vi "Hatch Controller.vi"(8 "error in":errorcluster) -> ()   [LabVIEW 2018]
doc: "This VI executes continuously carrying out the current operation and responding to updates or new operations. It will often contain the timing or control code that is difficult to place directly in TeleOp. This VI generally opens all sensors and motors and isolates the rest of the robot code from knowing how the operations are carried out."
uses:
  <vilib>/Rock Robotics/WPI/Framework/Completion Status.ctl
  Hatch Setpoints.ctl
  Hatch Operations.ctl
  <vilib>/Rock Robotics/WPI/Solenoid/WPI_SolenoidChannel.ctl
  <vilib>/Rock Robotics/WPI/Solenoid/WPI_SolenoidValue.ctl
  <vilib>/Rock Robotics/WPI/Solenoid/WPI_SolenoidOpenDouble.vi
  <vilib>/Rock Robotics/WPI/Solenoid/WPI_SolenoidSetEnum.vi
  <vilib>/Rock Robotics/Network Tables/NT Write Boolean.vi
panel:
  in  "Interactive Values":T1
  out "Current\nCmd":string
  in  "Buttons":cluster{"Execute Cmd":bool, "Abort Cmd":bool}
  out "Command Timing":cluster{"Start Time (ms)":u32, "Iterations":i32}
  out "Status":T3
  # "Tip: It may be helpful to observe inputs and sensor values.\nYou may also want to display tuning or debugging controls."
  # "Interactive Command: You may fill in the settings for a command\nand schedule it with the Execute button. You can observe and abort\nany command while fine tuning the code for the controller."
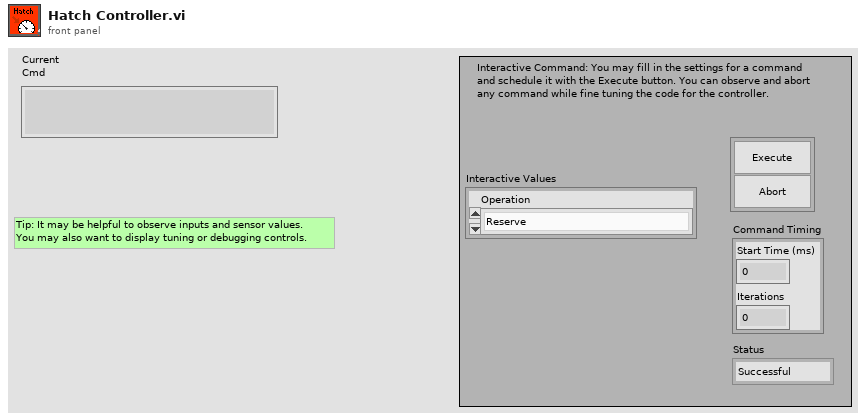
[diagram p1: front panel]
types:
  T1 = typedef "Hatch Setpoints.ctl" = cluster{"Operation":T2}
  T2 = typedef "Hatch Operations.ctl" = enum16{"Reserve", "Read Current", "Hatch Gripper In", "Hatch Gripper Out", "Extend Gripper Plate", "Retract Gripper Plate", "Retract HAB Piston", "Extend HAB Piston"}
  T3 = typedef "Completion Status.ctl" = enum16{"Successful", "Aborted", "Incomplete"}
  T4 = typedef "WPI_SolenoidChannel.ctl" = enum8{"Solenoid 0", "Solenoid 1", "Solenoid 2", "Solenoid 3", "Solenoid 4", "Solenoid 5", "Solenoid 6", "Solenoid 7", "Invalid"}
  T5 = typedef "WPI_SolenoidDevRef.ctl" = cluster{"DevStatus":errorcluster, "Pneumatics Control Module":u8, "Forward Solenoid Channel":T4, "Reverse Solenoid Channel":T4}
  T6 = typedef "Command Status Info.ctl" = cluster{"Name":string, "Status":T3, "notifier out":T7}
  T7 = typedef "Completion Notifier.ctl" = refnum<notifier>
  T8 = cluster{"Current Command":T1, "Command Timing":cluster{"Start Time (ms)":u32, "Iterations":i32}, "Command Arguments":cluster{"Command Info":T6, "Description":string, "Default Command":T1, "queue out":refnum<queue>, "Subsystem Name":string}}
  T9 = typedef "WPI_SolenoidValue.ctl" = enum16{"Off", "On", "Forward", "Reverse"}
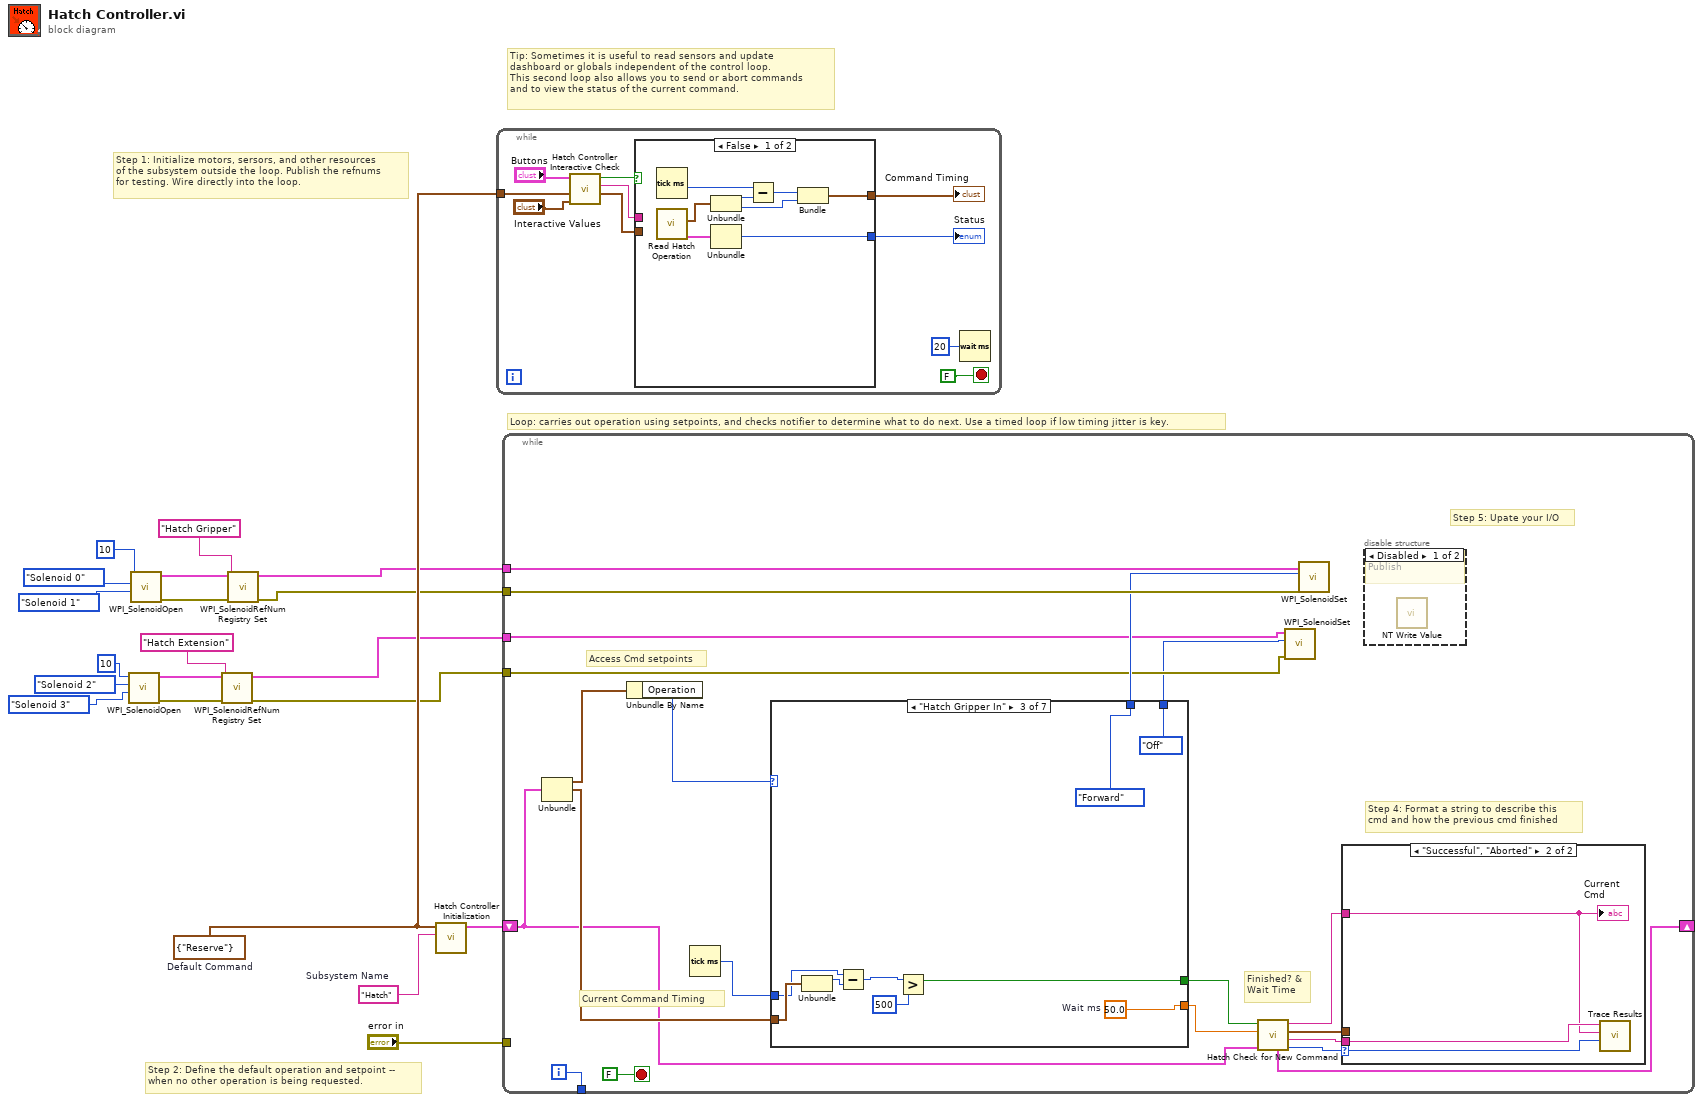
[diagram p0: block diagram]
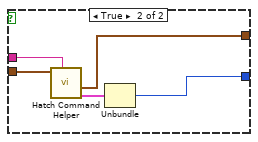
[diagram p2: hidden frame]
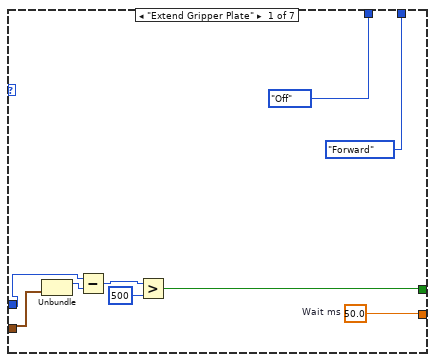
[diagram p5: hidden frame]
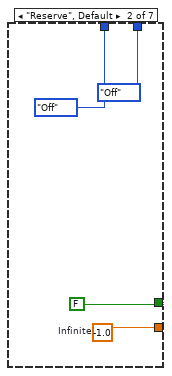
[diagram p6: hidden frame]
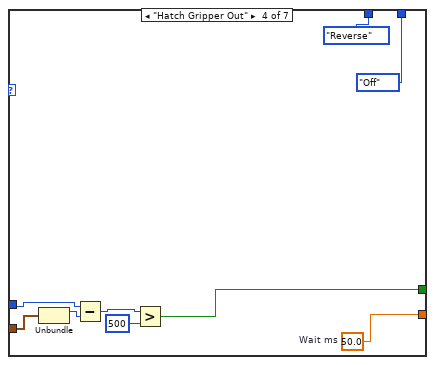
[diagram p7: hidden frame]
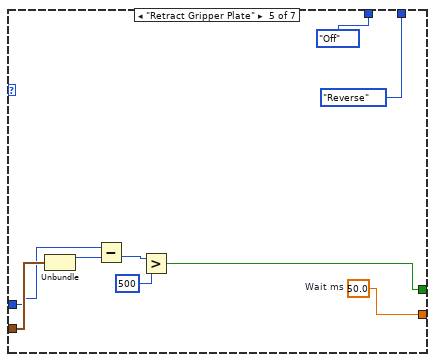
[diagram p8: hidden frame]
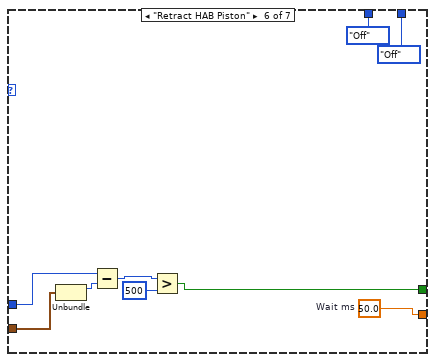
[diagram p9: hidden frame]
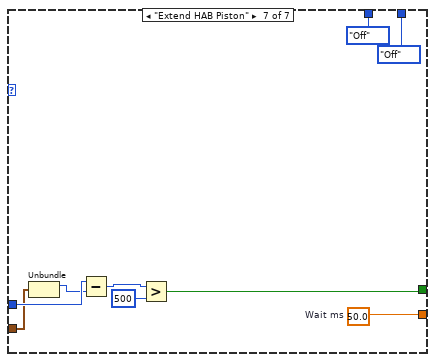
[diagram p10: hidden frame]
diagram:
  w17 = T1 {"Operation"=enum."Reserve"}  # Default Command
  w18 = "Hatch"  # Subsystem Name
  # "Tip: Sometimes it is useful to read sensors and update\ndashboard or globals independent of the control loop.\nThis second loop also allows you to send or abort commands\nand to view the status of the current command."
  # "Step 2: Define the default operation and setpoint --\nwhen no other operation is being requested."
  # "Step 1: Initialize motors, sersors, and other resources\nof the subsystem outside the loop. Publish the refnums\nfor testing. Wire directly into the loop."
  # "Loop: carries out operation using setpoints, and checks notifier to determine what to do next. Use a timed loop if low timing jitter is key."
  n1 = call-poly <vilib>:"WPI_SolenoidOpen.vi"("Reverse Solenoid Channel"=WPI_SolenoidChannel."Solenoid 3", "Forward Solenoid Channel"=WPI_SolenoidChannel."Solenoid 2", "Pneumatics Control Module (0)"=u8 10) -> ("error out"=w5:errorcluster, "SolenoidDevRef"=w4:T5)  [unwired: 7 in]
  n2 = call-poly <vilib>:"WPI_SolenoidOpen.vi"("Reverse Solenoid Channel"=WPI_SolenoidChannel."Solenoid 1", "Forward Solenoid Channel"=WPI_SolenoidChannel."Solenoid 0", "Pneumatics Control Module (0)"=u8 10) -> ("error out"=w13:errorcluster, "SolenoidDevRef"=w14:T5)  [unwired: 7 in]
  n3 = call <vilib>:"WPI_SolenoidRefNum Registry Set.vi"("error in (no error)"=w5, "refnum name"="Hatch Extension", "SolenoidDevRef"=w4) -> ("error out"=w2:errorcluster, "SolenoidDevRef"=w3:T5)  [unwired: 7 in]
  n4 = call <vilib>:"WPI_SolenoidRefNum Registry Set.vi"("error in (no error)"=w13, "refnum name"="Hatch Gripper", "SolenoidDevRef"=w14) -> ("error out"=w12:errorcluster, "SolenoidDevRef"=w11:T5)  [unwired: 7 in]
  n5 = call "Hatch Controller Initialization.vi"("Subsystem Name"=w18, "Default Command"=w17) -> ("Current Command"=w19:T8)  [unwired: 9 in]
  n6 = while {
    tunnel: w17 -> [w27]
    stop <- FALSE stop-if-true
    n7 = call "Hatch Controller Interactive Check.vi"("Interactive Command in"="Interactive Values", "Default Command"=w27, "Buttons"="Buttons") -> ("Interactive Command out"=w24:T1, "Trace String"=w25:string, "Schedule"=w26:bool)  [unwired: 6 in]
    n8 = case shown="False" w26 {
      tunnel: [w38 w43] -> w23
      tunnel: w24 -> [_ w41]
      tunnel: [w34 w39] -> w22
      tunnel: w25 -> [_ w42]
      frame False {
        n9 = Tick Count (ms)() -> (millisecond timer value=w33:u32)
        n10 = call "Read Hatch Operation.vi"() -> ("Command Info"=w32:T6, "Command Timing"=w31:cluster{"Start Time (ms)":u32, "Iterations":i32})  [unwired: 9 in, 1 out]
        n11 = Unbundle(w31) -> ("Start Time (ms)"=w37:u32, "Iterations"=w35:i32)
        n12 = Unbundle(w32) -> ("Status"=w38:T3)  [unwired: 2 out]
        n13 = Subtract(x=w33, y=w37) -> (x-y=w36:u32)
        n14 = Bundle(w36, "Iterations"=w35) -> (w34:cluster{u32, "Iterations":i32})  [unwired: 1 in]
      }
      frame True {
        n15 = call "Hatch Command Helper.vi"("Description"=w42, "SubSystem Data"=w41) -> ("Command Info Out"=w40:T6, "Command Timing"=w39:cluster{"Start Time (ms)":u32, "Iterations":i32})  [unwired: 7 in, 1 out]
        n16 = Unbundle(w40) -> ("Status"=w43:T3)  [unwired: 2 out]
      }
    }
    "Status" <- w23
    "Command Timing" <- w22
    n17 = Wait (ms)(milliseconds to wait=u32 20) -> ()  [unwired: 1 out]
  }
  n18 = while {
    shift-right: [w57] -> _
    shift-left: w19 -> [w50]
    tunnel: [w62] -> _
    tunnel: "error in" -> [_]
    tunnel: w12 -> [w49]
    tunnel: w11 -> [w48]
    tunnel: w3 -> [w46]
    tunnel: w2 -> [w45]
    i -> [w62]
    stop <- FALSE stop-if-true
    # "Step 5: Upate your I/O"
    # "Step 4: Format a string to describe this\ncmd and how the previous cmd finished"
    # "Current Command Timing"
    # "Access Cmd setpoints"
    # "Finished? &\nWait Time"
    n19 = Unbundle(w50) -> ("Current Command"=w61:T1, "Command Timing"=w58:cluster{"Start Time (ms)":u32, "Iterations":i32})  [unwired: 1 out]
    n20 = Unbundle By Name(w61) -> ("Operation"=w60:T2)
    n21 = Tick Count (ms)() -> (millisecond timer value=w59:u32)
    n22 = case shown="\"Hatch Gripper In\"" w60 {
      tunnel: [w69 w79 w83 w92 w102 w110 w119] -> w55
      tunnel: [w70 FALSE ("ignore previous (F)") w82 w91 w101 w111 w120] -> w56
      tunnel: w58 -> [w71 _ w86 w95 w100 w108 w117]
      tunnel: w59 -> [w72 _ w84 w94 w98 w109 w118]
      tunnel: [WPI_SolenoidValue."Off" ("Value") WPI_SolenoidValue."Off" ("Value") WPI_SolenoidValue."Forward" ("Value") WPI_SolenoidValue."Reverse" ("Value") WPI_SolenoidValue."Off" ("Value") WPI_SolenoidValue."Off" ("Value") WPI_SolenoidValue."Off" ("Value")] -> w47
      tunnel: [WPI_SolenoidValue."Forward" ("Value") WPI_SolenoidValue."Off" ("Value") WPI_SolenoidValue."Off" ("Value") WPI_SolenoidValue."Off" ("Value") WPI_SolenoidValue."Reverse" ("Value") WPI_SolenoidValue."Off" ("Value") WPI_SolenoidValue."Off" ("Value")] -> w44
      frame "Extend Gripper Plate" {
        w69 = 50.0  # Wait ms
        n23 = Unbundle(w71) -> ("Start Time (ms)"=w74:u32)  [unwired: 1 out]
        n24 = Subtract(x=w72, y=w74) -> (x-y=w75:u32)
        n25 = Greater?(x=w75, y=u32 500) -> (0:w70:bool)
      }
      frame "Reserve", Default {
        w79 = -1.0  # Infinite
      }
      frame "Hatch Gripper In" {
        w83 = 50.0  # Wait ms
        n26 = Unbundle(w86) -> ("Start Time (ms)"=w85:u32)  [unwired: 1 out]
        n27 = Subtract(x=w84, y=w85) -> (x-y=w88:u32)
        n28 = Greater?(x=w88, y=u32 500) -> (0:w82:bool)
      }
      frame "Hatch Gripper Out" {
        w92 = 50.0  # Wait ms
        n29 = Unbundle(w95) -> ("Start Time (ms)"=w93:u32)  [unwired: 1 out]
        n30 = Subtract(x=w94, y=w93) -> (x-y=w97:u32)
        n31 = Greater?(x=w97, y=u32 500) -> (0:w91:bool)
      }
      frame "Retract Gripper Plate" {
        w102 = 50.0  # Wait ms
        n32 = Unbundle(w100) -> ("Start Time (ms)"=w99:u32)  [unwired: 1 out]
        n33 = Subtract(x=w98, y=w99) -> (x-y=w104:u32)
        n34 = Greater?(x=w104, y=u32 500) -> (0:w101:bool)
      }
      frame "Retract HAB Piston" {
        w110 = 50.0  # Wait ms
        n35 = Unbundle(w108) -> ("Start Time (ms)"=w107:u32)  [unwired: 1 out]
        n36 = Subtract(x=w109, y=w107) -> (x-y=w113:u32)
        n37 = Greater?(x=w113, y=u32 500) -> (0:w111:bool)
      }
      frame "Extend HAB Piston" {
        w119 = 50.0  # Wait ms
        n38 = Unbundle(w117) -> ("Start Time (ms)"=w116:u32)  [unwired: 1 out]
        n39 = Subtract(x=w118, y=w116) -> (x-y=w122:u32)
        n40 = Greater?(x=w122, y=u32 500) -> (0:w120:bool)
      }
    }
    n41 = call "Hatch Check for New Command.vi"("Current Command"=w50, "Wait time (ms)"=w55, "Finished?"=w56) -> ("Completion"=w51:T3, "Subsystem Name"=w52:string, "Current Command"=w53:T1, "Initial Trace String"=w54:string, "NextCommand"=w57:T8)  [unwired: 4 in]
    n42 = call-poly <vilib>:"WPI_SolenoidSet.vi"("error in (no error)"=w45, "Value"=w44, "SolenoidDevRef"=w46) -> ()  [unwired: 7 in, 2 out]
    n43 = call-poly <vilib>:"WPI_SolenoidSet.vi"("error in (no error)"=w49, "Value"=w47, "SolenoidDevRef"=w48) -> ()  [unwired: 7 in, 2 out]
    n44 = case shown="\"Successful\", \"Aborted\"" w51 {
      selector: w51 -> [_ w66]
      tunnel: w54 -> [_ w64]
      tunnel: w53 -> [_ _]
      tunnel: w52 -> [_ w65]
      frame "Incomplete", Default {
        # "Continuing current command"
      }
      frame "Successful", "Aborted" {
        # "Report and setup for next command"
        n45 = call <vilib>:"Trace Results.vi"("Status of previous command"=w66, "Description"=w64, "Subsystem"=w65) -> ()  [unwired: 9 in]
        "Current\nCmd" <- w64
      }
    }
    n46 = disable-structure shown="Disabled" {
      frame Disabled {
        # "Publish"
        n47 = call-poly <vilib>:"NT Write Value.vi"() -> ()  [unwired: 11 in, 1 out]
      }
      frame Enabled {
      }
    }
  }
